vi "Start DI.vi"(0 "reference in":refnum<class "DI.lvclass">, 5 "error in (no error)":errorcluster) -> (14 "reference out":refnum<class "DI.lvclass">, 19 "error out":errorcluster)   [LabVIEW 2017, in "DI.lvclass"]
uses:
  DI.lvclass
  utils/DI_Read.vi
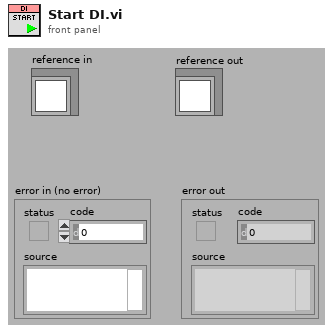
[diagram p1: front panel]
types:
  T1 = typedef "DI.lvclass/ObjectAttributes.ctl" = cluster{"DI Task":refnum<k21>, "DI Status":bool[], "DI Module Names (NI-Max Name)":string[], "Number of Channels Per DI Module":i32[], "Number of DI Modules":u32, "Number of Total DI Channels":u32, "DI On/Off Status":bool, "DO VI Reference":refnum<vi>}
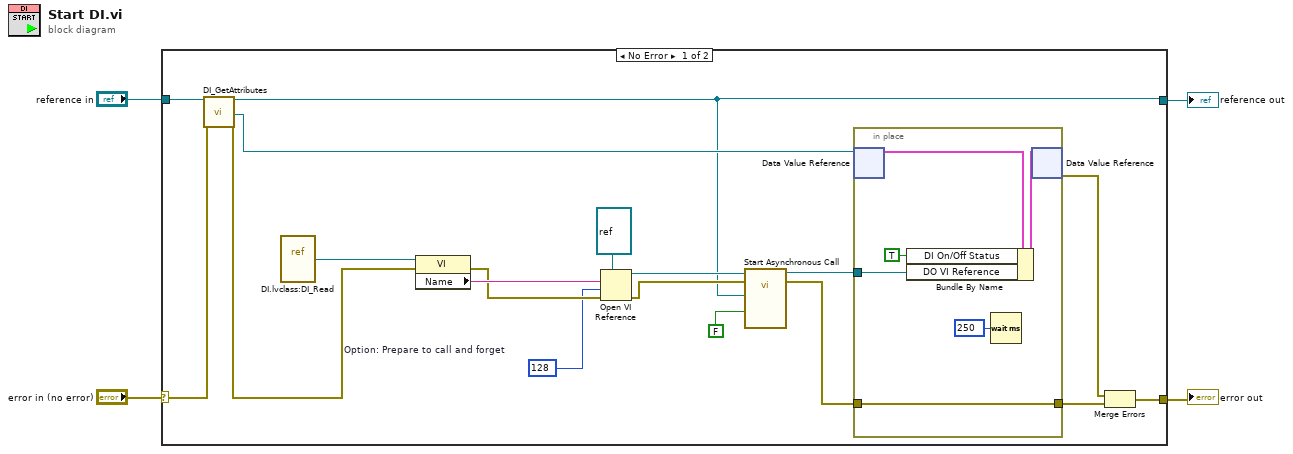
[diagram p0: block diagram]
diagram:
  n1 = case shown="No Error" "error in (no error)" {
    selector: "error in (no error)" -> [w21 w30]
    tunnel: [w19 w30] -> w3
    tunnel: [w5 w29] -> w1
    tunnel: "reference in" -> [w22 w29]
    frame No Error {
      w13 = 128  # Option: Prepare to call and forget
      n2 = call "DI_GetAttributes.vi"("reference in"=w22, "error in (no error)"=w21) -> ("reference out"=w5:refnum<class "DI.lvclass">, "DataRef"=w18:refnum<data-value>, "error out"=w12:errorcluster)  [unwired: 14 in, 1 out]
      n3 = vi-ref "DI.lvclass:DI_Read.vi"() -> (w15:refnum<vi>)
      n4 = property class="VI"(reference=w15, error in=w12) -> (error out=w14:errorcluster, "Name"=w16:string)  [unwired: 1 out]
      n5 = Open VI Reference(type specifier VI Refnum (for type only)=refnum<vi> refnum, vi path=w16, options=w13, error in (no error)=w14) -> (vi reference=w10:refnum<vi>, error out=w9:errorcluster)  [unwired: 2 in]
      n6 = call-by-ref "Start Asynchronous Call"(reference=w10, error in=w9, "Stop DI"=FALSE ("Stop Timer"), "reference in"=w5) -> (reference out=w8:refnum<vi>, error out=w7:errorcluster)  [unwired: 8 in, 2 out]
      n7 = in-place {
        in-place-border: w7 -> [w26]
        in-place-border: [w26] -> w17
        in-place-border: w8 -> [w24]
        n8 = in-place-dvr #1(w18) -> (w27:T1)  [unwired: 1 out]
        n9 = Bundle By Name(cluster=w27, "DI On/Off Status"=TRUE, "DO VI Reference"=w24) -> (w28:T1)
        n10 = Wait (ms)(milliseconds to wait=u32 250) -> ()  [unwired: 1 out]
        n11 = in-place-dvr #1(w28) -> (w20:errorcluster)  [unwired: 1 out]
      }
      n12 = Merge Errors(w20, w17) -> (w19:errorcluster)
    }
    frame Error {
    }
  }
  "error out" <- w3
  "reference out" <- w1
